vi "test-ControllerUtil.vi"(8 "error in (no error)":errorcluster) -> (0 "error out":errorcluster, 3 "All Tests Passed":bool)   [LabVIEW 2019]
uses:
  <vilib>/Rock Robotics/WPI/ThirdParty/JAS_Junk/TrajLib/Trajectory_Library.lvlib
panel:
  out "T1  = -20":dbl
  out "T0  = -20":dbl
  # "Controller Util -- Modulus Error test..."
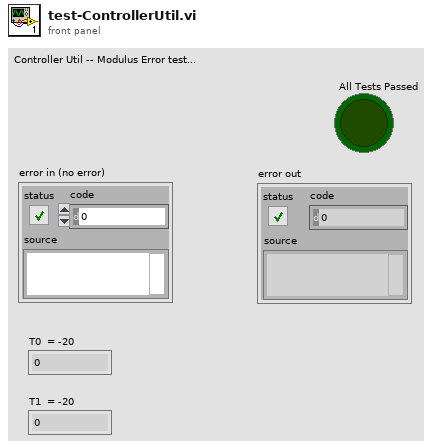
[diagram p1: front panel]
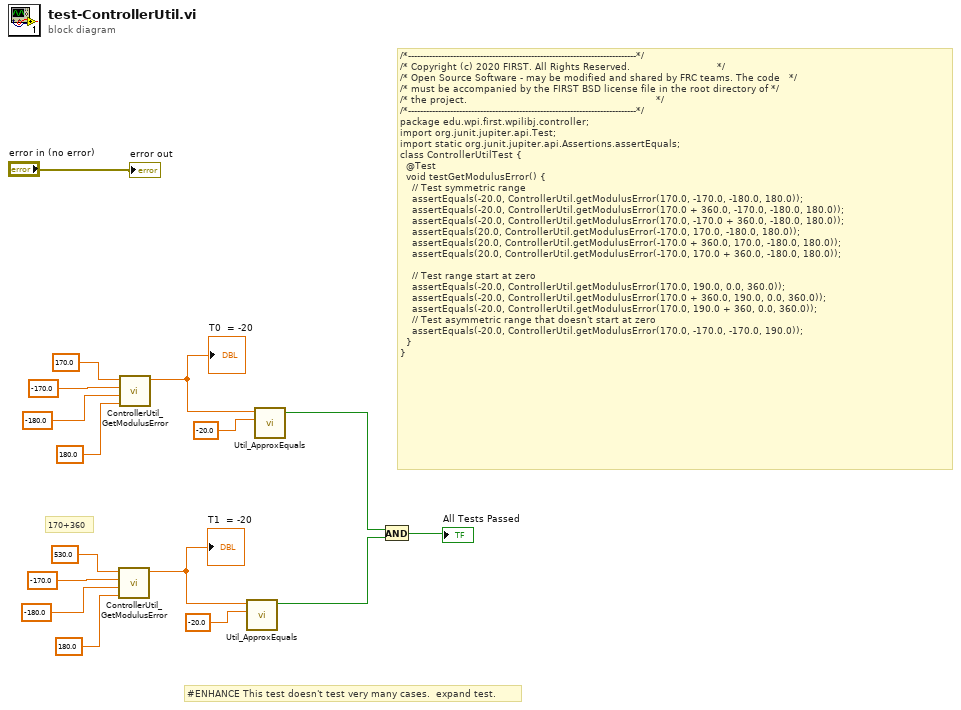
[diagram p0: block diagram]
diagram:
  # "#ENHANCE This test doesn't test very many cases.  expand test."
  # "170+360"
  # "/*----------------------------------------------------------------------------*/\n/* Copyright (c) 2020 FIRST. All Rights Reserved.                             */\n/* Open Source Software - may be modified and shared by FRC teams. The code   */\n/* must be accompanied by the FIRST BSD license file in the root directory of */\n/* the project.                                                               */\n/*----------------------------------------------------------------------------*/\npackage edu.wpi.first.wpilibj.controller;\nimport org.junit.jupiter.api.Test;\nimport static org.junit.jupiter.api.Assertions.assertEquals;\nclass ControllerUtilTest {\n  @Test\n  void testGetModulusError() {\n    // Test symmetric range\n    assertEquals(-20.0, ControllerUtil.getModulusError(170.0, -170.0, -180.0, 180.0));\n    assertEquals(-20.0, ControllerUtil.getModulusError(170.0 + 360.0, -170.0, -180.0, 180.0));\n    assertEquals(-20.0, ControllerUtil.getModulusError(170.0, -170.0 + 360.0, -180.0, 180.0));\n    assertEquals(20.0, ControllerUtil.getModulusError(-170.0, 170.0, -180.0, 180.0));\n    assertEquals(20.0, ControllerUtil.getModulusError(-170.0 + 360.0, 170.0, -180.0, 180.0));\n    assertEquals(20.0, ControllerUtil.getModulusError(-170.0, 170.0 + 360.0, -180.0, 180.0));\n\n    // Test range start at zero\n    assertEquals(-20.0, ControllerUtil.getModulusError(170.0, 190.0, 0.0, 360.0));\n    assertEquals(-20.0, ControllerUtil.getModulusError(170.0 + 360.0, 190.0, 0.0, 360.0));\n    assertEquals(-20.0, ControllerUtil.getModulusError(170.0, 190.0 + 360, 0.0, 360.0));\n    // Test asymmetric range that doesn't start at zero\n    assertEquals(-20.0, ControllerUtil.getModulusError(170.0, -170.0, -170.0, 190.0));\n  }\n}"
  n1 = call <vilib>:"ControllerUtil_GetModulusError.vi"("Maximum_Input"=180.0, "Minimum_Input"=-180.0, "Measurerment(PV)"=-170.0, "Reference(SP)"=530.0) -> ("Error"=w5:dbl)  [unwired: 7 in]
  "T1  = -20" <- w5
  n2 = call <vilib>:"ControllerUtil_GetModulusError.vi"("Maximum_Input"=180.0, "Minimum_Input"=-180.0, "Measurerment(PV)"=-170.0, "Reference(SP)"=170.0) -> ("Error"=w8:dbl)  [unwired: 7 in]
  "T0  = -20" <- w8
  n3 = call <vilib>:"Util_ApproxEquals.vi"("Value 2"=-20.0, "Value 1"=w5) -> ("ApproxEquals"=w2:bool)  [unwired: 9 in]
  n4 = call <vilib>:"Util_ApproxEquals.vi"("Value 2"=-20.0, "Value 1"=w8) -> ("ApproxEquals"=w3:bool)  [unwired: 9 in]
  n5 = And(x=w3, y=w2) -> (x .and. y?=→"All Tests Passed":bool)
  "error out" <- "error in (no error)"
